vi "Select one Image Array.vi"(1 "Previous Images (F)":T1[](array[typedef]), 2 "New Images (T)":T1[](array[typedef]), 4 "Image to use":bool) -> (6 "Selected Images":T1[](array[typedef]))   [LabVIEW 2021, in "Image.lvlib"]
uses:
  <vilib>/vision/Image Controls.llb/IMAQ Image.ctl
  Image.lvlib
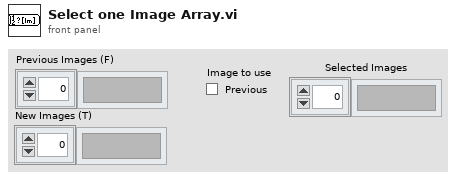
[diagram p1: front panel]
types:
  T1 = typedef "IMAQ Image.ctl" = refnum<image>
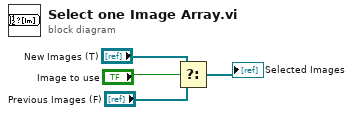
[diagram p0: block diagram]
diagram:
  n1 = Select(t="New Images (T)", s="Image to use", f="Previous Images (F)") -> (s? t:f=→"Selected Images":T1[])
